vi "Read Camera Status.vi"(8 "error in (no error)":errorcluster, 11 "CCDCamera in":refnum<class "Simulated_CCD_Camera.lvclass">) -> (0 "error out":errorcluster, 2 "Camera Status":T1, 3 "CCDCamera out":refnum<class "Simulated_CCD_Camera.lvclass">)   [LabVIEW 2018, in "Simulated_CCD_Camera.lvclass"]
uses:
  Simulated_CCD_Camera.lvclass
  Simulated_CCD_Camera.lvclass/Simulated_CCD_Camera.ctl
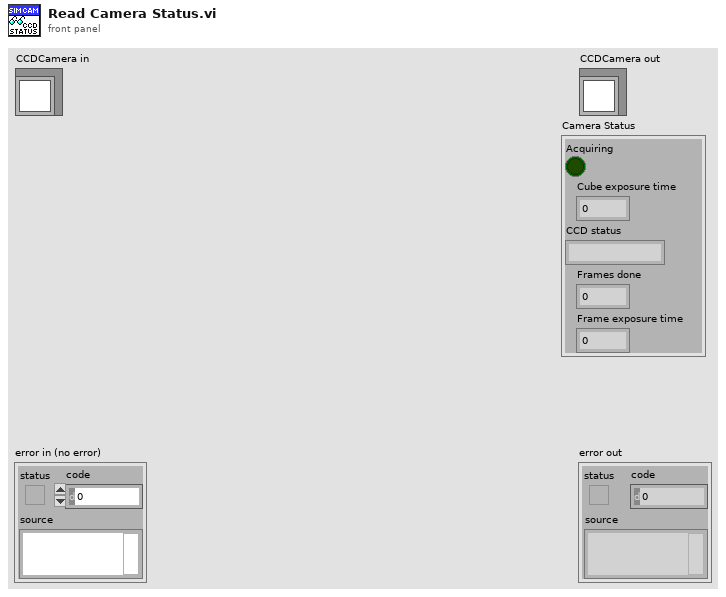
[diagram p1: front panel]
types:
  T1 = cluster{"Acquiring":bool, "Cube exposure time":sgl, "CCD status":string, "Frames done":u32, "Frame exposure time":dbl}
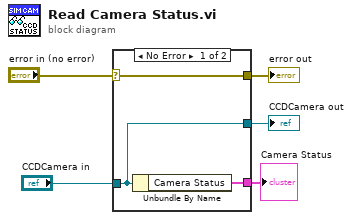
[diagram p0: block diagram]
diagram:
  n1 = case shown="No Error" "error in (no error)" {
    selector: "error in (no error)" -> [w7 w10]
    tunnel: [w7 w10] -> w5
    tunnel: [w8 w9] -> w4
    tunnel: "CCDCamera in" -> [w8 w9]
    tunnel: [w6 _] -> w1
    frame No Error {
      n2 = Unbundle By Name(w8) -> ("Camera Status"=w6:T1)
    }
    frame Error {
    }
  }
  "error out" <- w5
  "CCDCamera out" <- w4
  "Camera Status" <- w1
